vi "GEA2 Commands Dishwasher Converter.vi"(10 "Data":u8[](array[numeric]), 11 "Dishwasher":T1) -> (2 "GEA2 Data":string[][](array[string]), 3 "Dishwasher Out":T1)   [LabVIEW 2016]
uses:
  Type Definitions/GEA2 Commands Dishwasher.ctl
panel:
  out "appended array":u16[](array[numeric])
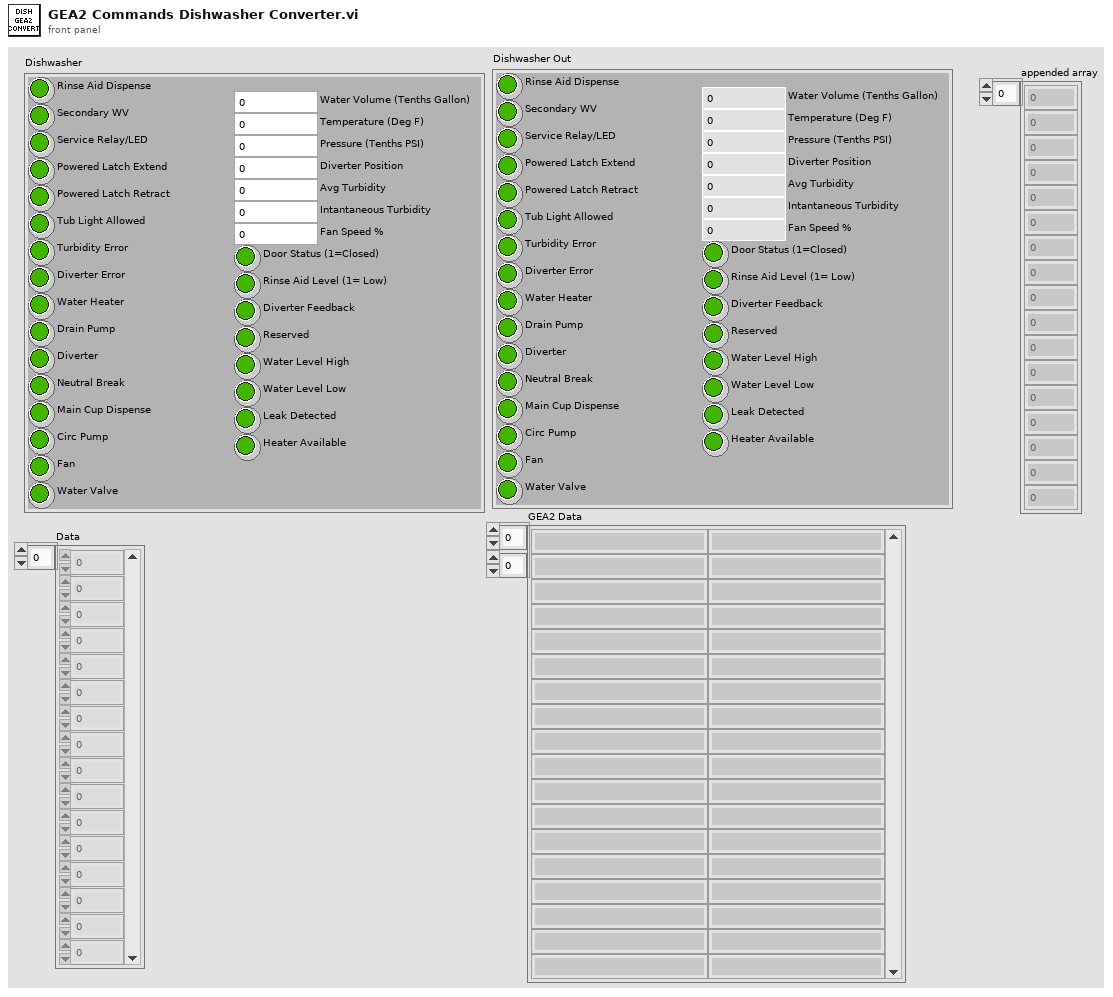
[diagram p1: front panel]
types:
  T1 = typedef "GEA2 Commands Dishwasher.ctl" = cluster{"Rinse Aid Dispense":bool, "Secondary WV":bool, "Diverter Error":bool, "Service Relay/LED":bool, "Powered Latch Extend":bool, "Powered Latch Retract":bool, "Tub Light Allowed":bool, "Turbidity Error":bool, "Water Heater":bool, "Drain Pump":bool, "Diverter":bool, "Neutral Break":bool, "Main Cup Dispense":bool, "Circ Pump":bool, "Fan":bool, "Water Valve":bool, "Water Volume (Tenths Gallon)":u8, "Temperature (Deg F)":u8, "Pressure (Tenths PSI)":u8, "Diverter Position":u8, "Avg Turbidity":u16, "Intantaneous Turbidity":u16, "Door Status (1=Closed)":bool, "Rinse Aid Level (1= Low)":bool, "Diverter Feedback":bool, "Reserved":bool, "Water Level High":bool, "Water Level Low":bool, "Leak Detected":bool, "Heater Available":bool, "Fan Speed %":u8}
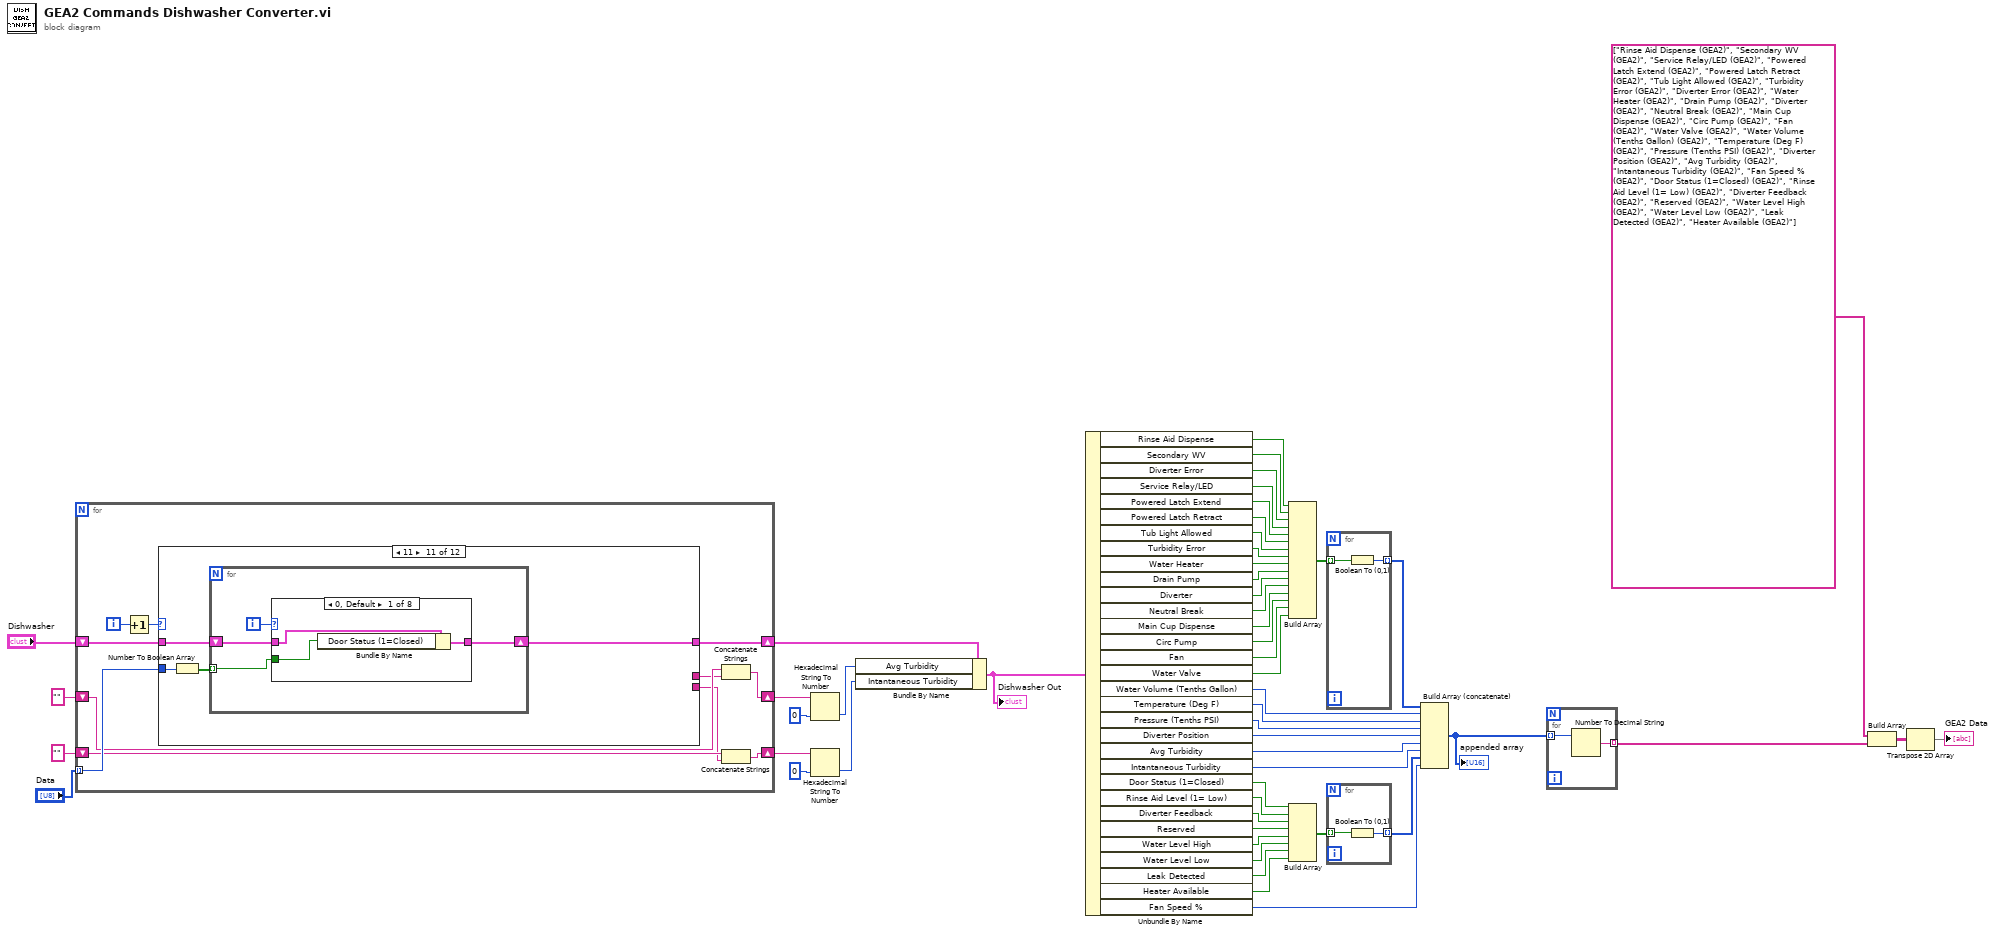
[diagram p0: block diagram]
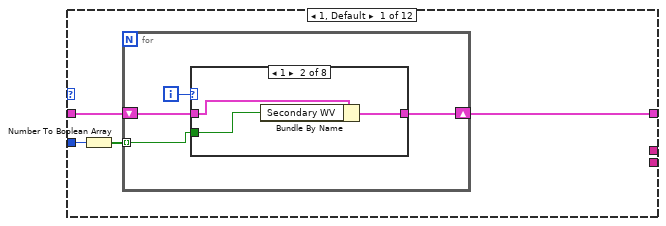
[diagram p2: hidden frame]
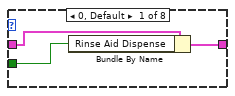
[diagram p3: hidden frame]
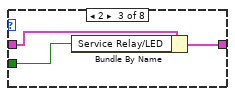
[diagram p4: hidden frame]
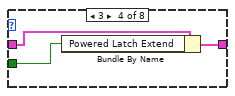
[diagram p5: hidden frame]
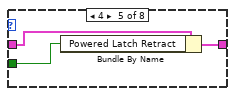
[diagram p6: hidden frame]
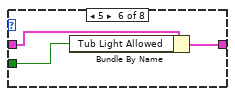
[diagram p7: hidden frame]
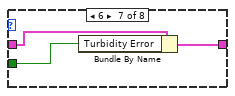
[diagram p8: hidden frame]
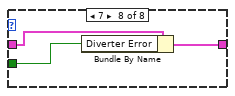
[diagram p9: hidden frame]
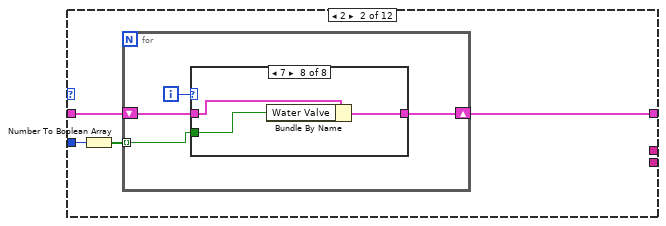
[diagram p10: hidden frame]
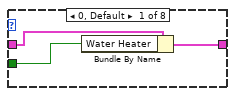
[diagram p11: hidden frame]
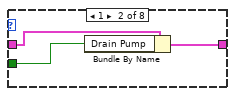
[diagram p12: hidden frame]
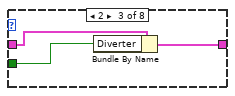
[diagram p13: hidden frame]
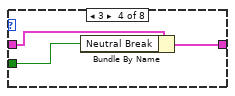
[diagram p14: hidden frame]
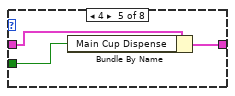
[diagram p15: hidden frame]
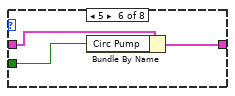
[diagram p16: hidden frame]
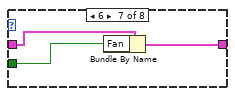
[diagram p17: hidden frame]
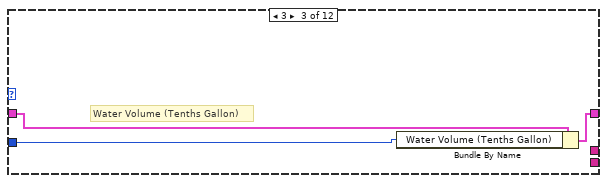
[diagram p18: hidden frame]
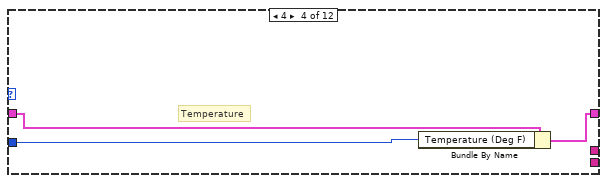
[diagram p19: hidden frame]
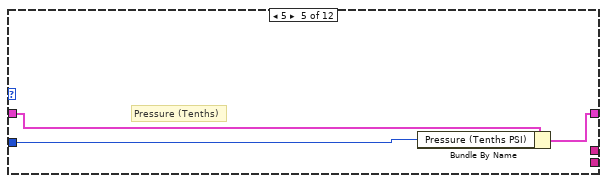
[diagram p20: hidden frame]
diagram:
  n1 = for {
    tunnel: "Data" -> [w63] mode=indexing
    shift-right: [w61] -> w45
    shift-left: "Dishwasher" -> [w60]
    shift-right: [w56] -> w48
    shift-left: "" -> [w58]
    shift-right: [w53] -> w52
    shift-left: "" -> [w55]
    i -> [w62]
    n2 = Increment(x=w62) -> (x+1=w59:i32)
    n3 = case shown="11" w59 {
      tunnel: w63 -> [w67 w97 w129 w131 w134 w137 w141 w145 w147 w150 w155 w184]
      tunnel: w60 -> [w66 w99 w130 w133 w136 w139 w142 w144 w148 w151 w153 w186]
      tunnel: [w65 w98 w128 w132 w135 w138 w142 w144 w148 w151 w152 w185] -> w61
      tunnel: [_ _ _ _ _ _ w140 w143 _ _ _ _] -> w57
      tunnel: [_ _ _ _ _ _ _ _ w146 w149 _ _] -> w54
      frame 1, Default {
        n4 = Number To Boolean Array(number=w67) -> (Boolean array=w64:bool[])
        n5 = for {
          shift-right: [w70] -> w65
          shift-left: w66 -> [w71]
          tunnel: w64 -> [w68] mode=indexing
          i -> [w69]
          n6 = case shown="1" w69 {
            tunnel: w71 -> [w74 w77 w80 w83 w86 w89 w92 w95]
            tunnel: [w73 w76 w79 w82 w85 w88 w91 w94] -> w70
            tunnel: w68 -> [w72 w75 w78 w81 w84 w87 w90 w93]
            frame 0, Default {
              n7 = Bundle By Name(cluster=w74, "Rinse Aid Dispense"=w72) -> (w73:T1)
            }
            frame 1 {
              n8 = Bundle By Name(cluster=w77, "Secondary WV"=w75) -> (w76:T1)
            }
            frame 2 {
              n9 = Bundle By Name(cluster=w80, "Service Relay/LED"=w78) -> (w79:T1)
            }
            frame 3 {
              n10 = Bundle By Name(cluster=w83, "Powered Latch Extend"=w81) -> (w82:T1)
            }
            frame 4 {
              n11 = Bundle By Name(cluster=w86, "Powered Latch Retract"=w84) -> (w85:T1)
            }
            frame 5 {
              n12 = Bundle By Name(cluster=w89, "Tub Light Allowed"=w87) -> (w88:T1)
            }
            frame 6 {
              n13 = Bundle By Name(cluster=w92, "Turbidity Error"=w90) -> (w91:T1)
            }
            frame 7 {
              n14 = Bundle By Name(cluster=w95, "Diverter Error"=w93) -> (w94:T1)
            }
          }
        }
      }
      frame 2 {
        n15 = Number To Boolean Array(number=w97) -> (Boolean array=w96:bool[])
        n16 = for {
          shift-right: [w102] -> w98
          shift-left: w99 -> [w103]
          tunnel: w96 -> [w100] mode=indexing
          i -> [w101]
          n17 = case shown="7" w101 {
            tunnel: w103 -> [w106 w109 w112 w115 w118 w121 w124 w127]
            tunnel: [w105 w108 w111 w114 w117 w120 w123 w126] -> w102
            tunnel: w100 -> [w104 w107 w110 w113 w116 w119 w122 w125]
            frame 0, Default {
              n18 = Bundle By Name(cluster=w106, "Water Heater"=w104) -> (w105:T1)
            }
            frame 1 {
              n19 = Bundle By Name(cluster=w109, "Drain Pump"=w107) -> (w108:T1)
            }
            frame 2 {
              n20 = Bundle By Name(cluster=w112, "Diverter"=w110) -> (w111:T1)
            }
            frame 3 {
              n21 = Bundle By Name(cluster=w115, "Neutral Break"=w113) -> (w114:T1)
            }
            frame 4 {
              n22 = Bundle By Name(cluster=w118, "Main Cup Dispense"=w116) -> (w117:T1)
            }
            frame 5 {
              n23 = Bundle By Name(cluster=w121, "Circ Pump"=w119) -> (w120:T1)
            }
            frame 6 {
              n24 = Bundle By Name(cluster=w124, "Fan"=w122) -> (w123:T1)
            }
            frame 7 {
              n25 = Bundle By Name(cluster=w127, "Water Valve"=w125) -> (w126:T1)
            }
          }
        }
      }
      frame 3 {
        # "Water Volume (Tenths Gallon)"
        n26 = Bundle By Name(cluster=w130, "Water Volume (Tenths Gallon)"=w129) -> (w128:T1)
      }
      frame 4 {
        # "Temperature"
        n27 = Bundle By Name(cluster=w133, "Temperature (Deg F)"=w131) -> (w132:T1)
      }
      frame 5 {
        # "Pressure (Tenths)"
        n28 = Bundle By Name(cluster=w136, "Pressure (Tenths PSI)"=w134) -> (w135:T1)
      }
      frame 6 {
        # "Diverter Position"
        n29 = Bundle By Name(cluster=w139, "Diverter Position"=w137) -> (w138:T1)
      }
      frame 7 {
        # "Average Turbidity MSB"
        n30 = Number To Hexadecimal String(2:w141) -> (0:w140:string)  [unwired: 1 in]
      }
      frame 8 {
        # "Average Turbidity LSB"
        n31 = Number To Hexadecimal String(2:w145) -> (0:w143:string)  [unwired: 1 in]
      }
      frame 9 {
        # "Intantaneous Turbidity (MSB)"
        n32 = Number To Hexadecimal String(2:w147) -> (0:w146:string)  [unwired: 1 in]
      }
      frame 10 {
        # "Instantaneous Turbidity (LSB)"
        n33 = Number To Hexadecimal String(2:w150) -> (0:w149:string)  [unwired: 1 in]
      }
      frame 11 {
        n34 = Number To Boolean Array(number=w155) -> (Boolean array=w154:bool[])
        n35 = for {
          shift-right: [w158] -> w152
          shift-left: w153 -> [w159]
          tunnel: w154 -> [w156] mode=indexing
          i -> [w157]
          n36 = case shown="0, Default" w157 {
            tunnel: w159 -> [w162 w165 w168 w171 w174 w177 w180 w183]
            tunnel: [w161 w164 w167 w170 w173 w176 w179 w182] -> w158
            tunnel: w156 -> [w160 w163 w166 w169 w172 w175 w178 w181]
            frame 0, Default {
              n37 = Bundle By Name(cluster=w162, "Door Status (1=Closed)"=w160) -> (w161:T1)
            }
            frame 1 {
              n38 = Bundle By Name(cluster=w165, "Rinse Aid Level (1= Low)"=w163) -> (w164:T1)
            }
            frame 2 {
              n39 = Bundle By Name(cluster=w168, "Diverter Feedback"=w166) -> (w167:T1)
            }
            frame 3 {
              n40 = Bundle By Name(cluster=w171, "Reserved"=w169) -> (w170:T1)
            }
            frame 4 {
              n41 = Bundle By Name(cluster=w174, "Water Level High"=w172) -> (w173:T1)
            }
            frame 5 {
              n42 = Bundle By Name(cluster=w177, "Water Level Low"=w175) -> (w176:T1)
            }
            frame 6 {
              n43 = Bundle By Name(cluster=w180, "Leak Detected"=w178) -> (w179:T1)
            }
            frame 7 {
              n44 = Bundle By Name(cluster=w183, "Heater Available"=w181) -> (w182:T1)
            }
          }
        }
      }
      frame 12 {
        # "Fan Speed %"
        n45 = Bundle By Name(cluster=w186, "Fan Speed %"=w184) -> (w185:T1)
      }
    }
    n46 = Concatenate Strings(w58, w57) -> (w56:string)
    n47 = Concatenate Strings(w55, w54) -> (w53:string)
  }
  n48 = Hexadecimal String To Number(string=w48, default (0uL)=u16 0 ("default (0 U32)")) -> (number=w44:u16)  [unwired: 1 in, 1 out]
  n49 = Hexadecimal String To Number(string=w52, default (0uL)=u16 0 ("default (0 U32)")) -> (number=w43:u16)  [unwired: 1 in, 1 out]
  n50 = Bundle By Name(cluster=w45, "Avg Turbidity"=w44, "Intantaneous Turbidity"=w43) -> (w41:T1)
  "Dishwasher Out" <- w41
  n51 = Unbundle By Name(w41) -> ("Rinse Aid Dispense"=w40:bool, "Secondary WV"=w39:bool, "Diverter Error"=w38:bool, "Service Relay/LED"=w37:bool, "Powered Latch Extend"=w36:bool, "Powered Latch Retract"=w35:bool, "Tub Light Allowed"=w34:bool, "Turbidity Error"=w33:bool, "Water Heater"=w32:bool, "Drain Pump"=w31:bool, "Diverter"=w30:bool, "Neutral Break"=w29:bool, "Main Cup Dispense"=w28:bool, "Circ Pump"=w27:bool, "Fan"=w26:bool, "Water Valve"=w25:bool, "Water Volume (Tenths Gallon)"=w13:u8, "Temperature (Deg F)"=w12:u8, "Pressure (Tenths PSI)"=w11:u8, "Diverter Position"=w10:u8, "Avg Turbidity"=w9:u16, "Intantaneous Turbidity"=w8:u16, "Door Status (1=Closed)"=w24:bool, "Rinse Aid Level (1= Low)"=w23:bool, "Diverter Feedback"=w22:bool, "Reserved"=w21:bool, "Water Level High"=w20:bool, "Water Level Low"=w19:bool, "Leak Detected"=w18:bool, "Heater Available"=w17:bool, "Fan Speed %"=w6:u8)
  n52 = Build Array(w40, w39, w38, w37, w36, w35, w34, w33, w32, w31, w30, w29, w28, w27, w26, w25) -> (w16:bool[])
  n53 = Build Array(w24, w23, w22, w21, w20, w19, w18, w17) -> (w15:bool[])
  n54 = for {
    tunnel: w16 -> [w188] mode=indexing
    tunnel: [w187] -> w14 mode=indexing
    n55 = Boolean To (0,1)(Boolean=w188) -> (0, 1=w187:i16)
  }
  n56 = for {
    tunnel: w15 -> [w190] mode=indexing
    tunnel: [w189] -> w7 mode=indexing
    n57 = Boolean To (0,1)(Boolean=w190) -> (0, 1=w189:i16)
  }
  n58 = Build Array (concatenate)(w14, w13, w12, w11, w10, w9, w8, w7, w6) -> (w5:u16[])
  "appended array" <- w5
  n59 = for {
    tunnel: w5 -> [w192] mode=indexing
    tunnel: [w191] -> w3 mode=indexing
    n60 = Number To Decimal String(number=w192) -> (decimal integer string=w191:string)  [unwired: 1 in]
  }
  n61 = Build Array(string[] ["Rinse Aid Dispense (GEA2)", "Secondary WV (GEA2)", "Service Relay/LED (GEA2)", "Powered Latch Extend (GEA2)", "Powered Latch Retract (GEA2)", "Tub Light Allowed (GEA2)", "Turbidity Error (GEA2)", "Diverter Error (GEA2)", "Water Heater (GEA2)", "Drain Pump (GEA2)", "Diverter (GEA2)", "Neutral Break (GEA2)", "Main Cup Dispense (GEA2)", "Circ Pump (GEA2)", "Fan (GEA2)", "Water Valve (GEA2)", "Water Volume (Tenths Gallon) (GEA2)", "Temperature (Deg F) (GEA2)", "Pressure (Tenths PSI) (GEA2)", "Diverter Position (GEA2)", "Avg Turbidity (GEA2)", "Intantaneous Turbidity (GEA2)", "Fan Speed % (GEA2)", "Door Status (1=Closed) (GEA2)", "Rinse Aid Level (1= Low) (GEA2)", "Diverter Feedback (GEA2)", "Reserved (GEA2)", "Water Level High (GEA2)", "Water Level Low (GEA2)", "Leak Detected (GEA2)", "Heater Available (GEA2)"] ("Headers"), w3) -> (w2:string[][])
  n62 = Transpose 2D Array(2D array=w2) -> (transposed array=→"GEA2 Data":string[][])
